vi "reporteword.vi"() -> ()   [LabVIEW 2016]
uses:
  <vilib>/addons/_office/_exclsub.llb/font.ctl
  <vilib>/addons/_office/word.llb/Word Easy Table (num).vi
  <vilib>/printing/ReportDocExtensions.llb/Append Front Panel Image to Report (path).vi
  <vilib>/printing/ReportDocExtensions.llb/Append VI Block Diagram to Report (path).vi
  <vilib>/Utility/NIReport.llb/NI_report.lvclass
  <vilib>/addons/_office/NI_ReportGenerationToolkit.lvlib
  <vilib>/Utility/NIReport.llb/NI_ReportGenerationCore.lvlib
panel:
  in  "report file path":path
  in  "VI":path
  out "Gauge":dbl(knob) scale=0.0..10.0
  out "XY Graph":cluster{"X":dbl, "Y":dbl}[](graph)
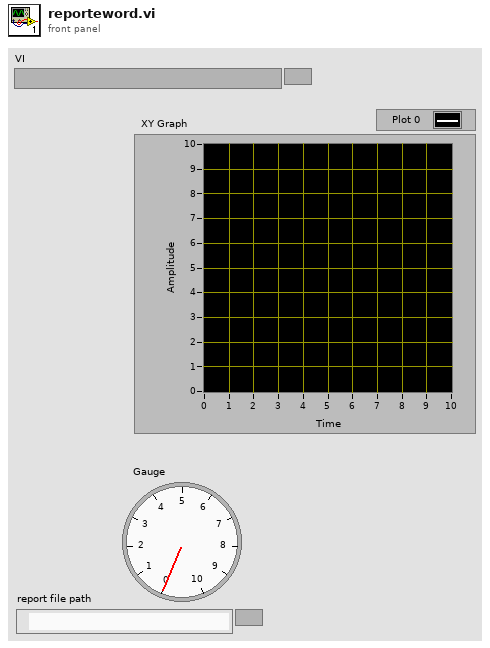
[diagram p1: front panel]
types:
  T1 = typedef "NI_ReportGenerationToolkit.lvlib/font.ctl" = cluster{"font name":string, "font size":dbl, "bold":u16, "italic":u16, "underline":u16, "strike through":u16, "font color":u32}
  T2 = enum16{"xlColumnClustered", "xlColumnStacked", "xlColumnStacked100", "xl3DColumnClustered", "xl3DColumnStacked", "xl3DColumnStacked100", "xlBarClustered", "xlBarStacked", "xlBarStacked100", "xl3DBarClustered", "xl3DBarStacked", "xl3DBarStacked100", "xlLineStacked", "xlLineStacked100", "xlLineMarkers", "xlLineMarkersStacked", "xlLineMarkersStacked100", "xlPieOfPie", "xlPieExploded", "xl3DPieExploded", "xlBarOfPie", "xlXYScatterSmooth", "xlXYScatterSmoothNoMarkers", "xlXYScatterLines", "xlXYScatterLinesNoMarkers", "xlAreaStacked", "xlAreaStacked100", "xl3DAreaStacked", "xl3DAreaStacked100", "xlDoughnutExploded", "xlRadarMarkers", "xlRadarFilled", "xlSurface", "xlSurfaceWireframe", "xlSurfaceTopView", "xlSurfaceTopViewWireframe", "xlBubble", "xlBubble3DEffect", "xlStockHLC", "xlStockOHLC", "xlStockVHLC", "xlStockVOHLC", "xlCylinderColClustered", "xlCylinderColStacked", "xlCylinderColStacked100", "xlCylinderBarClustered", "xlCylinderBarStacked", "xlCylinderBarStacked100", "xlCylinderCol", "xlConeColClustered", "xlConeColStacked", "xlConeColStacked100", "xlConeBarClustered", "xlConeBarStacked", "xlConeBarStacked100", "xlConeCol", "xlPyramidColClustered", "xlPyramidColStacked", "xlPyramidColStacked100", "xlPyramidBarClustered", "xlPyramidBarStacked", "xlPyramidBarStacked100", "xlPyramidCol", "xl3DColumn", "xlLine", "xl3DLine", "xl3DPie", "xlPie", "xlXYScatter", "xl3DArea", "xlArea", "xlDoughnut", "xlRadar"}
  T3 = enum16{"Standard Report", "HTML", "Word", "Excel"}
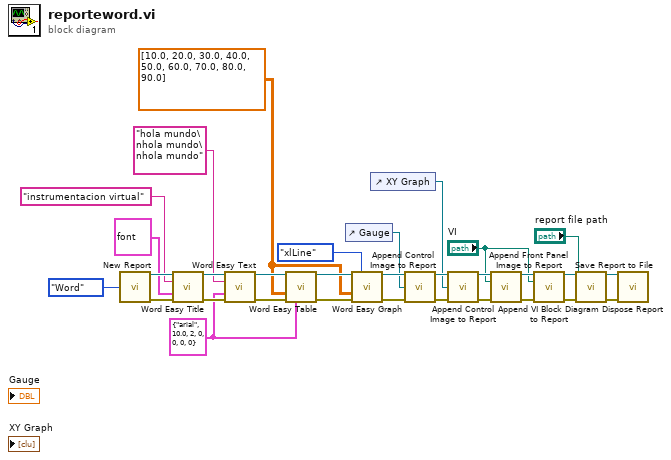
[diagram p0: block diagram]
diagram:
  w17 = T1 {"font name"="arial", "font size"=10.0, "bold"=2, "italic"=0, "underline"=0, "strike through"=0, "font color"=0} ("font")
  w20 = dbl[][] [[10.0, 20.0, 30.0], [40.0, 50.0, 60.0], [70.0, 80.0, 90.0]] ("text data")
  n1 = call <vilib>:"New Report.vi"("report type"=T3."Word") -> ("report out"=w30:refnum<class "NI_report.lvclass">, "error out"=w29:errorcluster)  [unwired: 13 in]
  n2 = call <vilib>:"Word Easy Title.vi"("report in"=w30, "title"="instrumentacion virtual", "font"=T1 {"font name"="impact", "font size"=36.0, "bold"=1, "italic"=0, "underline"=0, "strike through"=0, "font color"=16716306}, "error in (no error)"=w29) -> ("report out"=w27:refnum<class "NI_report.lvclass">, "error out"=w26:errorcluster)  [unwired: 9 in, 1 out]
  n3 = call <vilib>:"Word Easy Text.vi"("report in"=w27, "text"="hola mundo\nhola mundo\nhola mundo", "font"=w17, "error in (no error)"=w26) -> ("report out"=w24:refnum<class "NI_report.lvclass">, "error out"=w23:errorcluster)  [unwired: 9 in, 1 out]
  n4 = call-poly <vilib>:"Word Easy Table.vi"("report in"=w24, "text data"=w20, "error in (no error)"=w23, "font"=w17) -> ("report out"=w22:refnum<class "NI_report.lvclass">, "error out"=w21:errorcluster)  [unwired: 9 in, 1 out]
  n5 = control-ref of="Gauge"() -> (w12:refnum<vi>)
  n6 = call <vilib>:"Word Easy Graph.vi"("report in"=w22, "graph type (col clustered)"=T2."xlLine", "data"=w20, "error in (no error)"=w21) -> ("report out"=w16:refnum<class "NI_report.lvclass">, "error out"=w15:errorcluster)  [unwired: 10 in]
  n7 = control-ref of="XY Graph"() -> (w11:refnum<vi>)
  n8 = call-dynamic "Append Control Image to Report.vi"("report in"=w16, "ctrl reference"=w12, "error in (no error)"=w15) -> ("report out"=w14:refnum<class "NI_report.lvclass">, "error out"=w13:errorcluster)  [unwired: 9 in, 2 out]
  n9 = call-dynamic "Append Control Image to Report.vi"("report in"=w14, "ctrl reference"=w11, "error in (no error)"=w13) -> ("report out"=w10:refnum<class "NI_report.lvclass">, "error out"=w9:errorcluster)  [unwired: 9 in, 2 out]
  n10 = call-poly <vilib>:"Append Front Panel Image to Report.vi"("report in"=w10, "VI"="VI", "error in (no error)"=w9) -> ("report out"=w8:refnum<class "NI_report.lvclass">, "error out"=w7:errorcluster)  [unwired: 8 in, 3 out]
  n11 = call-poly <vilib>:"Append VI Block Diagram to Report.vi"("report in"=w8, "VI"="VI", "error in (no error)"=w7) -> ("report out"=w5:refnum<class "NI_report.lvclass">, "error out"=w4:errorcluster)  [unwired: 8 in, 3 out]
  n12 = call-dynamic "Save Report to File.vi"("report in"=w5, "report file path"="report file path", "error in (no error)"=w4) -> ("report out"=w3:refnum<class "NI_report.lvclass">, "error out"=w2:errorcluster)  [unwired: 11 in]
  n13 = call-dynamic "Dispose Report.vi"("report in"=w3, "error in (no error)"=w2) -> ()  [unwired: 13 in, 1 out]
